vi "Write DAT (2D).vi"(4 "Append (0=F)":i32, 6 "Comments":string, 8 "error in":errorcluster, 9 "Data":dbl[][](array[numeric]), 10 "Headers":string[](array[string]), 11 "path":path) -> (0 "error out":errorcluster, 3 "new file path":path)   [LabVIEW 2020, in "Data.DAT.lvclass"]
uses:
  Data.DAT.lvclass
  <vilib>/Utility/file.llb/Write Delimited Spreadsheet (DBL).vi
  <vilib>/Utility/file.llb/Write Delimited Spreadsheet (string).vi
panel:
  out "appended array":string[][](array[string])
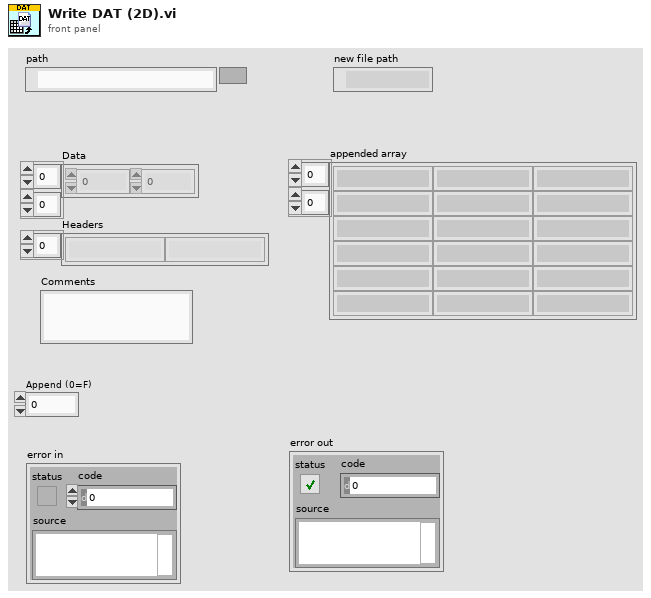
[diagram p1: front panel]
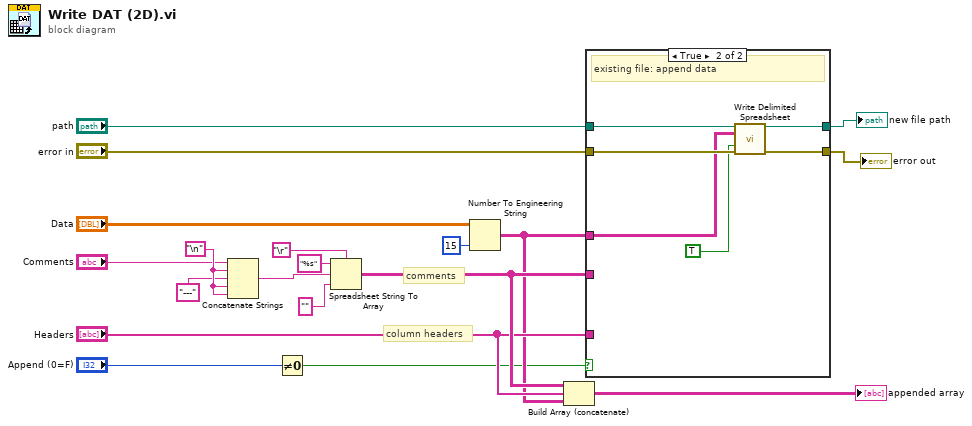
[diagram p0: block diagram]
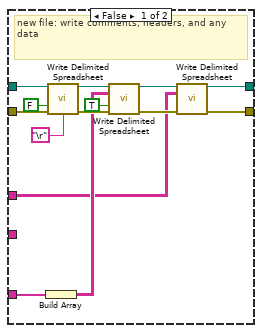
[diagram p2: hidden frame]
diagram:
  w12 = "\n"
  # "comments"
  # "column headers"
  n1 = Concatenate Strings("Comments", w12, "---" ("string"), w12, w12) -> (w13:string)
  n2 = Not Equal To 0?(x="Append (0=F)") -> (x != 0?=w1:bool)
  n3 = Spreadsheet String To Array(delimiter (Tab)="\r", format string="%s", spreadsheet string=w13, array type (2D Dbl)="") -> (array=w5:string[][])
  n4 = Number To Engineering String(2:i16 15 ("precision (6)"), 4:"Data") -> (0:w3:string[][])  [unwired: 2 out]
  n5 = Build Array (concatenate)(w5, "Headers", w3) -> (→"appended array":string[][])
  n6 = case shown="True" w1 {
    tunnel: [w21 w37] -> w7
    tunnel: "path" -> [w33 w39]
    tunnel: "error in" -> [w32 w38]
    tunnel: [w22 w36] -> w8
    tunnel: w3 -> [w20 w35]
    tunnel: "Headers" -> [w25 _]
    tunnel: w5 -> [_ _]
    frame False {
      # "new file: write comments, headers, and any data"
      n7 = Build Array(w25) -> (w26:string[][])
      n8 = call-poly <vilib>:"Write Delimited Spreadsheet.vi"("file path (dialog if empty)"=w33, "append to file? (new file:F)"=FALSE, "error in (no error)"=w32, "delimiter (\\t)"="\r") -> ("new file path (Not A Path if cancelled)"=w30:path, "error out"=w31:errorcluster)  [unwired: 10 in]
      n9 = call-poly <vilib>:"Write Delimited Spreadsheet.vi"("file path (dialog if empty)"=w30, "2D data"=w26, "append to file? (new file:F)"=TRUE, "error in (no error)"=w31) -> ("new file path (Not A Path if cancelled)"=w23:path, "error out"=w24:errorcluster)  [unwired: 10 in]
      n10 = call-poly <vilib>:"Write Delimited Spreadsheet.vi"("file path (dialog if empty)"=w23, "2D data"=w20, "error in (no error)"=w24) -> ("new file path (Not A Path if cancelled)"=w21:path, "error out"=w22:errorcluster)  [unwired: 11 in]
    }
    frame True {
      # "existing file: append data"
      n11 = call-poly <vilib>:"Write Delimited Spreadsheet.vi"("file path (dialog if empty)"=w39, "2D data"=w35, "append to file? (new file:F)"=TRUE, "error in (no error)"=w38) -> ("new file path (Not A Path if cancelled)"=w37:path, "error out"=w36:errorcluster)  [unwired: 10 in]
    }
  }
  "new file path" <- w7
  "error out" <- w8
